vi "엔코드 출력.vi"() -> ()   [LabVIEW 2014]
uses:
  <vilib>/DAQmx/create/channels.llb/DAQmx Create Channel (CI-Position-Angular Encoder).vi
  <vilib>/DAQmx/read.llb/DAQmx Read (Counter DBL 1Chan 1Samp).vi
panel:
  out "data":dbl caption="데이터" format="%0.2f"
  in  "정지":bool
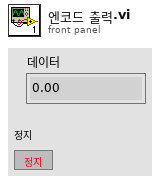
[diagram p1: front panel]
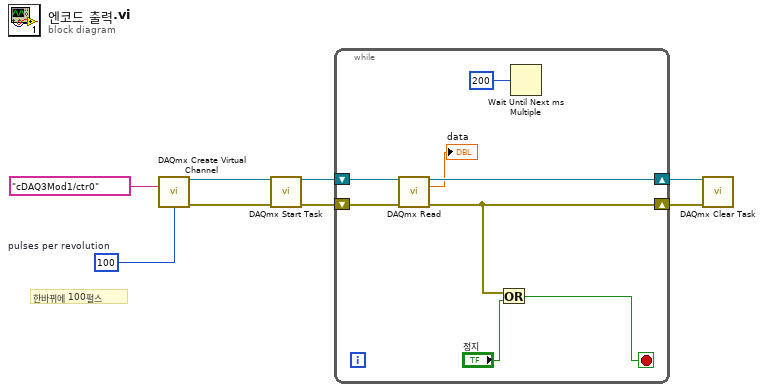
[diagram p0: block diagram]
diagram:
  w7 = u32 100  # pulses per revolution
  # "한바뀌에 100펄스"
  n1 = call-poly <vilib>:"DAQmx Create Virtual Channel.vi"("counter"=tag "cDAQ3Mod1/ctr0", "pulses per revolution"=w7) -> ("task out"=w6:refnum<k21>, "error out"=w5:errorcluster)  [unwired: 12 in]
  n2 = call <vilib>:"DAQmx Start Task.vi"("task/channels in"=w6, "error in"=w5) -> ("task out"=w4:refnum<k21>, "error out"=w3:errorcluster)  [unwired: 12 in]
  n3 = while {
    shift-right: [w14] -> w2
    shift-left: w4 -> [w16]
    shift-right: [w12] -> w1
    shift-left: w3 -> [w15]
    stop <- w10 stop-if-true
    n4 = call-poly <vilib>:"DAQmx Read.vi"("task/channels in"=w16, "error in"=w15) -> ("task out"=w14:refnum<k21>, "data"=→"data":dbl, "error out"=w12:errorcluster)  [unwired: 11 in]
    n5 = Or(x=w12, y="정지") -> (x .or. y?=w10:bool)
    n6 = Wait Until Next ms Multiple(millisecond multiple=u32 200 ("ms 배수")) -> ()  [unwired: 1 out]
  }
  n7 = call <vilib>:"DAQmx Clear Task.vi"("task in"=w2, "error in"=w1) -> ()  [unwired: 13 in, 1 out]
